vi "DFD Plot Pole-Zero.vi"(5 "output option":u16(ring) items=["Auto", "Floating-Point Only", "Fixed-Point Only"], 8 "error in (no error)":errorcluster, 10 "upper half plane only":bool=TRUE, 11 "filter in":T2={"mSRate_Fs"=1.0, "mSRate_Version"="2.0", "mSRate_Comments"="", "mSRate_OrgCoef"={"type"=enum."Undefined", "gain"=1.0, "coef a (k)"=[], "coef b (v)"=[]}, "mSRate_CurCoef"={"type"=enum."Undefined", "gain"=1.0, "coef a (k)"=[], "coef b (v)"=[]}, "mSRate_Quantized?"=FALSE, "mSRate_QCoef"={"type"=enum."Undefined", "gain"=1.0, "coef a (k)"=[], "coef b (v)"=[]}, "mSRate_QSettings"=[], "mSRate_Order"=0, "mSRate_Scaling"={"mSRate_ScaleByPowerOf2?"=FALSE, "mSRate_ScaleType"=enum."No Norm"}} {"mSRate_QSettings"."source" items=["Coef a/k"=0, "Coef b/v"=7, "Input"=1, "Output"=2, "Multiplicand"=3, "Product"=4, "Sum"=5, "Delay"=6, "Gain"=8]}) -> (0 "error out":errorcluster, 2 "Z-Plane":T1, 3 "filter out":T2={"mSRate_Fs"=1.0, "mSRate_Version"="2.0", "mSRate_Comments"="", "mSRate_OrgCoef"={"type"=enum."Undefined", "gain"=1.0, "coef a (k)"=[], "coef b (v)"=[]}, "mSRate_CurCoef"={"type"=enum."Undefined", "gain"=1.0, "coef a (k)"=[], "coef b (v)"=[]}, "mSRate_Quantized?"=FALSE, "mSRate_QCoef"={"type"=enum."Undefined", "gain"=1.0, "coef a (k)"=[], "coef b (v)"=[]}, "mSRate_QSettings"=[], "mSRate_Order"=0, "mSRate_Scaling"={"mSRate_ScaleByPowerOf2?"=FALSE, "mSRate_ScaleType"=enum."No Norm"}} {"mSRate_QSettings"."source" items=["Coef a/k"=0, "Coef b/v"=7, "Input"=1, "Output"=2, "Multiplicand"=3, "Product"=4, "Sum"=5, "Delay"=6, "Gain"=8]})   [LabVIEW 2017, in "NI_DigFilterLicensed.lvlib"]
doc: "Plots the poles and zeroes of a filter in the z-plane."
uses:
  <vilib>/addons/Digital Filter Design/NI_DigFilterLicensed.lvlib
  <vilib>/addons/Digital Filter Design/_Objects.llb/DFD Filter Obj.ctl
  <vilib>/addons/Digital Filter Design/_Objects.llb/DFD Filter Coef.ctl
  <vilib>/addons/Digital Filter Design/_Objects.llb/DFD Filter Structure Type Selector.ctl
  <vilib>/addons/Digital Filter Design/_Objects.llb/dfd_Internal Quantization Settings.ctl
  <vilib>/addons/Digital Filter Design/_Objects.llb/dfd_Internal Quantization Srcs.ctl
  <vilib>/addons/Digital Filter Design/_Objects.llb/DFD Coef Norm Type.ctl
  <vilib>/addons/Digital Filter Design/_Objects.llb/DFD Pole-Zero Plot.ctl
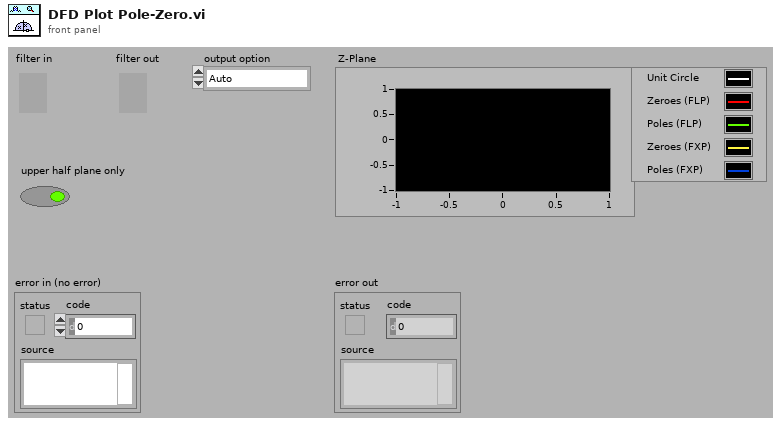
[diagram p1: front panel]
types:
  T1 = typedef "NI_DigFilterLicensed.lvlib/DFD Pole-Zero Plot.ctl" = cluster{dbl[], dbl[]}[]
  T2 = typedef "NI_DigFilterLicensed.lvlib/DFD Filter Obj.ctl" = cluster{"mSRate_Fs":dbl, "mSRate_Version":string, "mSRate_Comments":string, "mSRate_OrgCoef":T3, "mSRate_CurCoef":T3, "mSRate_Quantized?":bool, "mSRate_QCoef":T3, "mSRate_QSettings":T5[], "mSRate_Order":i32, "mSRate_Scaling":cluster{"mSRate_ScaleByPowerOf2?":bool, "mSRate_ScaleType":T7}}
  T3 = typedef "NI_DigFilterLicensed.lvlib/DFD Filter Coef.ctl" = cluster{"type":T4, "gain":dbl, "coef a (k)":dbl[], "coef b (v)":dbl[]}
  T4 = typedef "NI_DigFilterLicensed.lvlib/DFD Filter Structure Type Selector.ctl" = enum16{"Undefined", "FIR Direct Form", "FIR Direct Form Transposed", "FIR Symmetric", "FIR Antisymmetric", "IIR Direct Form I", "IIR Direct Form I Transposed", "IIR Direct Form II", "IIR Direct Form II Transposed", "IIR Cascaded Second Order Sections Form I", "IIR Cascaded Second Order Sections Form I Transposed", "IIR Cascaded Second Order Sections Form II", "IIR Cascaded Second Order Sections Form II Transposed", "Lattice Allpass (basic sections)", "Lattice Allpass (one multiplier sections)", "Lattice Allpass (normalized sections)", "Lattice AR (basic sections)", "Lattice AR (one multiplier sections)", "Lattice AR (normalized sections)", "Lattice MA (minimum phase)", "Lattice MA (maximum phase)", "Lattice ARMA (basic sections)", "Lattice ARMA (one multiplier sections)", "Lattice ARMA (normalized sections)"}
  T5 = typedef "NI_DigFilterLicensed.lvlib/dfd_Internal Quantization Settings.ctl" = cluster{"source":T6, "wl":i16, "iwl":i16, "overflow mode":enum16{"Saturation", "Wrap"}, "rounding mode":enum16{"Nearest", "Truncation"}, "signed?":bool}
  T6 = typedef "NI_DigFilterLicensed.lvlib/dfd_Internal Quantization Srcs.ctl" = u16
  T7 = typedef "NI_DigFilterLicensed.lvlib/DFD Coef Norm Type.ctl" = enum16{"No Norm", "Time Domain 1-Norm", "Time Domain 2-Norm", "Time Domain Inf-Norm"}
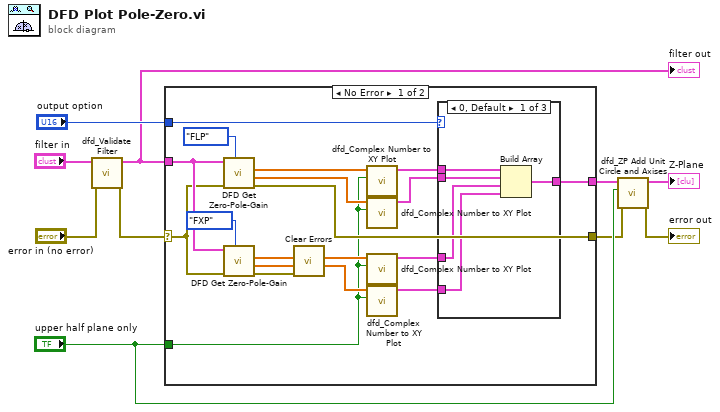
[diagram p0: block diagram]
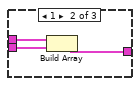
[diagram p2: hidden frame]
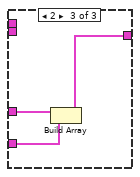
[diagram p3: hidden frame]
diagram:
  n1 = call <vilib>:"dfd_Validate Filter.vi"("error in (no error)"="error in (no error)", "filter in"="filter in") -> ("error out"=w1:errorcluster, "filter out"=w3:T2)  [unwired: 1 in, 7 out]
  "filter out" <- w3
  n2 = case shown="No Error" w1 {
    selector: w1 -> [w14 w39]
    tunnel: [w27 w39] -> w7
    tunnel: w3 -> [w15 _]
    tunnel: [w25 _] -> w10
    tunnel: "upper half plane only" -> [w16 _]
    tunnel: "output option" -> [w13 _]
    frame No Error {
      n3 = call <vilib>:"DFD Get Zero-Pole-Gain.vi"("type (FLP)"=enum16{"FLP", "FXP"}."FLP", "error in (no error)"=w14, "filter in"=w15) -> ("error out"=w27:errorcluster, "poles"=w22:cdb[], "zeroes"=w21:cdb[])  [unwired: 6 out]
      n4 = call <vilib>:"DFD Get Zero-Pole-Gain.vi"("type (FLP)"=enum16{"FLP", "FXP"}."FXP", "error in (no error)"=w14, "filter in"=w15) -> ("error out"=w26:errorcluster, "poles"=w24:cdb[], "zeroes"=w23:cdb[])  [unwired: 6 out]
      n5 = call <vilib>:"Clear Errors.vi"("error in (no error)"=w26) -> ()  [unwired: 1 in, 6 out]
      n6 = call <vilib>:"dfd_Complex Number to XY Plot.vi"("upper half plane only"=w16, "complex numbers"=w21) -> ("XY plot"=w20:cluster{dbl[], dbl[]})  [unwired: 9 out]
      n7 = call <vilib>:"dfd_Complex Number to XY Plot.vi"("upper half plane only"=w16, "complex numbers"=w22) -> ("XY plot"=w19:cluster{dbl[], dbl[]})  [unwired: 9 out]
      n8 = call <vilib>:"dfd_Complex Number to XY Plot.vi"("upper half plane only"=w16, "complex numbers"=w23) -> ("XY plot"=w18:cluster{dbl[], dbl[]})  [unwired: 9 out]
      n9 = call <vilib>:"dfd_Complex Number to XY Plot.vi"("upper half plane only"=w16, "complex numbers"=w24) -> ("XY plot"=w17:cluster{dbl[], dbl[]})  [unwired: 9 out]
      n10 = case shown="0, Default" w13 {
        tunnel: [w32 w33 w38] -> w25
        tunnel: w20 -> [w31 w35 _]
        tunnel: w19 -> [w30 w34 _]
        tunnel: w18 -> [w29 _ w37]
        tunnel: w17 -> [w28 _ w36]
        frame 0, Default {
          n11 = Build Array(w31, w30, w29, w28) -> (w32:cluster{dbl[], dbl[]}[])
        }
        frame 1 {
          n12 = Build Array(w35, w34) -> (w33:cluster{dbl[], dbl[]}[])
        }
        frame 2 {
          n13 = Build Array(w37, w36) -> (w38:cluster{dbl[], dbl[]}[])
        }
      }
    }
    frame Error {
    }
  }
  n14 = call <vilib>:"dfd_ZP Add Unit Circle and Axises.vi"("error in (no error)"=w7, "upper half plane only"="upper half plane only", "zero pole plot in"=w10) -> ("error out"=→"error out":errorcluster, "zero pole plot out"=→"Z-Plane":cluster{dbl[], dbl[]}[])  [unwired: 7 out]
